vi "VCS_CleanUp.vi"(5 "Error In":errorcluster) -> (19 "Error Out":errorcluster)   [LabVIEW 2023, in "VCS.lvclass"]
uses:
  VCS.lvclass
  VCS.lvclass/VCS.ctl
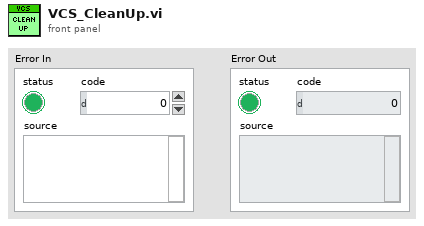
[diagram p1: front panel]
types:
  T1 = typedef "G4BaseTemplate_Singleton_6x8x6.lvclass/ObjectAttributes.ctl" = cluster{"Attribute1":dbl}
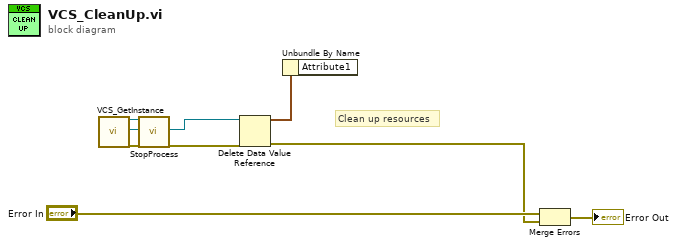
[diagram p0: block diagram]
diagram:
  # "Clean up resources"
  n1 = call "VCS_GetInstance.vi"() -> ("reference out"=w3:refnum<class "VCS.lvclass">, "DVRRefOut"=w5:refnum<data-value>, "Error Out"=w2:errorcluster)  [unwired: 15 in, 2 out]
  n2 = call "StopProcess.vi"("reference in"=w3, "Error In"=w2) -> ("Error Out"=w1:errorcluster)  [unwired: 16 in, 1 out]
  n3 = Delete Data Value Reference(data value reference=w5, error in=w1) -> (data value=w4:T1, error out=w6:errorcluster)
  n4 = Unbundle By Name(w4) -> ()  [unwired: 1 out]
  n5 = Merge Errors("Error In", w6) -> (→"Error Out":errorcluster)
